vi "Set Progress Window Progress.vi"(8 "error in (no error)":errorcluster, 10 "Progress":dbl, 11 "DVRs in":T1) -> (0 "error out":errorcluster, 3 "DVRs out":T1)   [LabVIEW 2019, in "Build Automation.lvlib"]
uses:
  Build Automation.lvlib
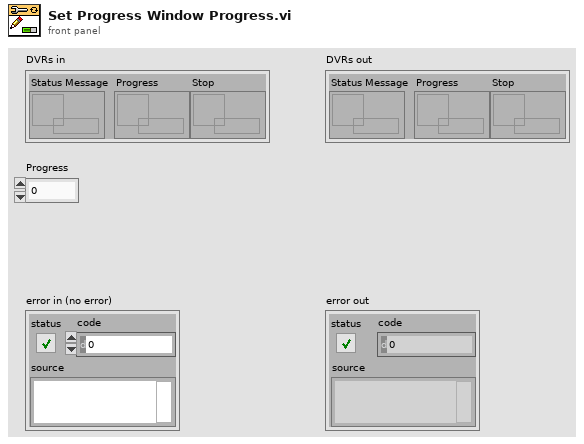
[diagram p1: front panel]
types:
  T1 = cluster{"Status Message":refnum<data-value>, "Progress":refnum<data-value>, "Stop":refnum<data-value>}
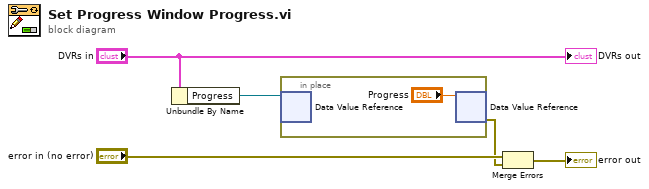
[diagram p0: block diagram]
diagram:
  n1 = Unbundle By Name("DVRs in") -> ("Progress"=w5:refnum<data-value>)
  n2 = in-place {
    n3 = in-place-dvr #1(w5) -> ()  [unwired: 2 out]
    n4 = in-place-dvr #1("Progress") -> (w3:errorcluster)  [unwired: 1 out]
  }
  n5 = Merge Errors("error in (no error)", w3) -> (→"error out":errorcluster)
  "DVRs out" <- "DVRs in"
